vi "retrieve_result_params.vi"(8 "error in (no error)":errorcluster, 11 "result_from_call in":refnum<class "result_from_call.lvclass">) -> (0 "error out":errorcluster, 2 "params":string, 3 "result_from_call out":refnum<class "result_from_call.lvclass">)   [LabVIEW 2015, in "result_from_call.lvclass"]
uses:
  result_from_call.lvclass
  result_from_call.lvclass/result_from_call.ctl
  result.lvclass
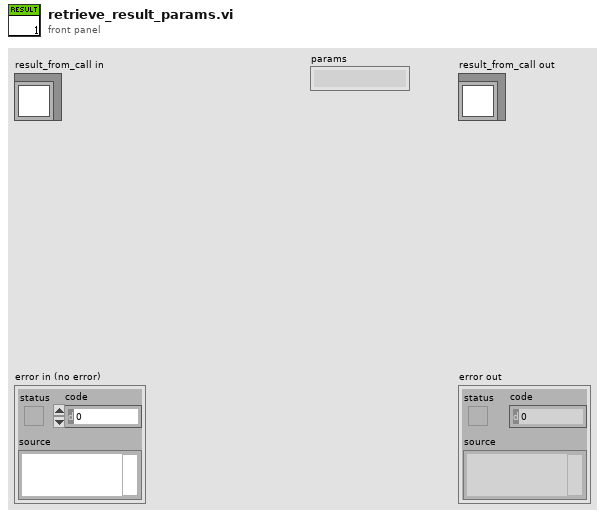
[diagram p1: front panel]
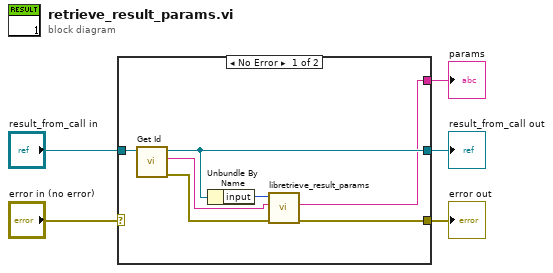
[diagram p0: block diagram]
diagram:
  n1 = case shown="No Error" "error in (no error)" {
    selector: "error in (no error)" -> [_ w14]
    tunnel: [w8 w14] -> w4
    tunnel: [w11 w13] -> w2
    tunnel: "result_from_call in" -> [w12 w13]
    tunnel: [w6 _] -> w1
    frame No Error {
      n2 = call "Get Id.vi"("result in"=w12) -> ("error out"=w7:errorcluster, "id"=w10:string, "result out"=w11:refnum<class "result_from_call.lvclass">)  [unwired: 8 in]
      n3 = Unbundle By Name(w11) -> ("input"=w9:i32)
      n4 = call "libretrieve_result_params.vi"("error in (no error)"=w7, "id"=w10, "input"=w9) -> ("error out"=w8:errorcluster, "params"=w6:string)  [unwired: 7 in]
    }
    frame Error {
    }
  }
  "error out" <- w4
  "result_from_call out" <- w2
  "params" <- w1
